vi "Rotate Box.vi"(9 "IMU":dbl) -> (2 "theta":dbl[](array[numeric]), 3 "r":dbl[](array[numeric]))   [LabVIEW 2020]
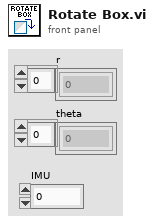
[diagram p1: front panel]
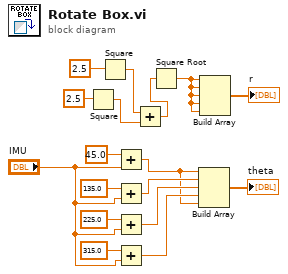
[diagram p0: block diagram]
diagram:
  n1 = Square(x=2.5) -> (x^2=w13:dbl)
  n2 = Square(x=2.5) -> (x^2=w5:dbl)
  n3 = Add(x=45.0 ("element"), y="IMU") -> (x+y=w2:dbl)
  n4 = Add(x=135.0 ("element"), y="IMU") -> (x+y=w8:dbl)
  n5 = Add(x=225.0 ("element"), y="IMU") -> (x+y=w7:dbl)
  n6 = Add(x=315.0 ("element"), y="IMU") -> (x+y=w6:dbl)
  n7 = Add(x=w5, y=w13) -> (x+y=w4:dbl)
  n8 = Square Root(x=w4) -> (sqrt(x)=w1:dbl)
  n9 = Build Array(w2, w8, w7, w6, w2) -> (→"theta":dbl[])
  n10 = Build Array(w1, w1, w1, w1, w1) -> (→"r":dbl[])
